vi "Init.vi"(8 "error in (no error)":errorcluster, 9 "Value JSON":string, 10 "Slot Name":string, 11 "Realm":T1) -> (0 "error out":errorcluster, 3 "SetPersistentData out":refnum<class "SetPersistentData.lvclass">)   [LabVIEW 2022 SP3, in "obs-websocket-lv.lvlib" / "SetPersistentData.lvclass"]
uses:
  SetPersistentData.lvclass
  SetPersistentData.lvclass/SetPersistentData.ctl
  Data Realm.ctl
  obs-websocket-lv.lvlib
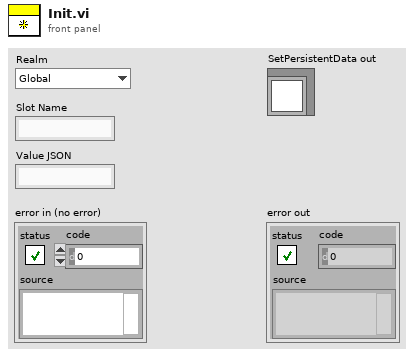
[diagram p1: front panel]
types:
  T1 = typedef "obs-websocket-lv.lvlib/Data Realm.ctl" = enum16{"Global", "Profile"}
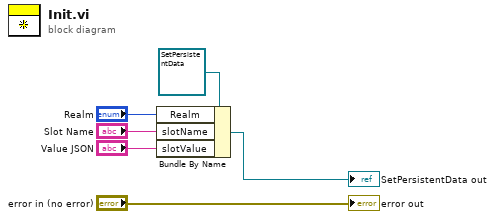
[diagram p0: block diagram]
diagram:
  n1 = Bundle By Name(cluster=refnum<class "SetPersistentData.lvclass"> refnum ("SetPersistentData in"), "Realm"="Realm", "slotName"="Slot Name", "slotValue"="Value JSON") -> (→"SetPersistentData out":refnum<class "SetPersistentData.lvclass">)
  "error out" <- "error in (no error)"
